vi "BinAndSaveWaveformsASCII.vi"(1 "transpose? (no:F)":bool, 4 "X step":dbl=0.10000000149011612 format="%.2f", 5 "format":string="%.6g", 6 "Deafault channel name prefix":string="CH", 7 "Channel name attribute":string="NI_ChannelName", 8 "error in":errorcluster, 9 "Save column names":bool, 10 "Y waveforms in":waveform(dbl)[](array[waveform]), 11 "file (use dialog)":path) -> (0 "error out":errorcluster)   [LabVIEW 2015]
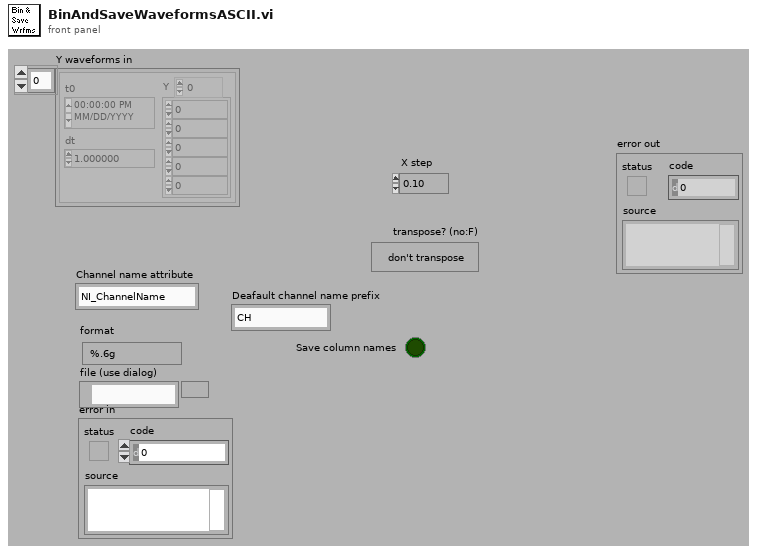
[diagram p1: front panel]
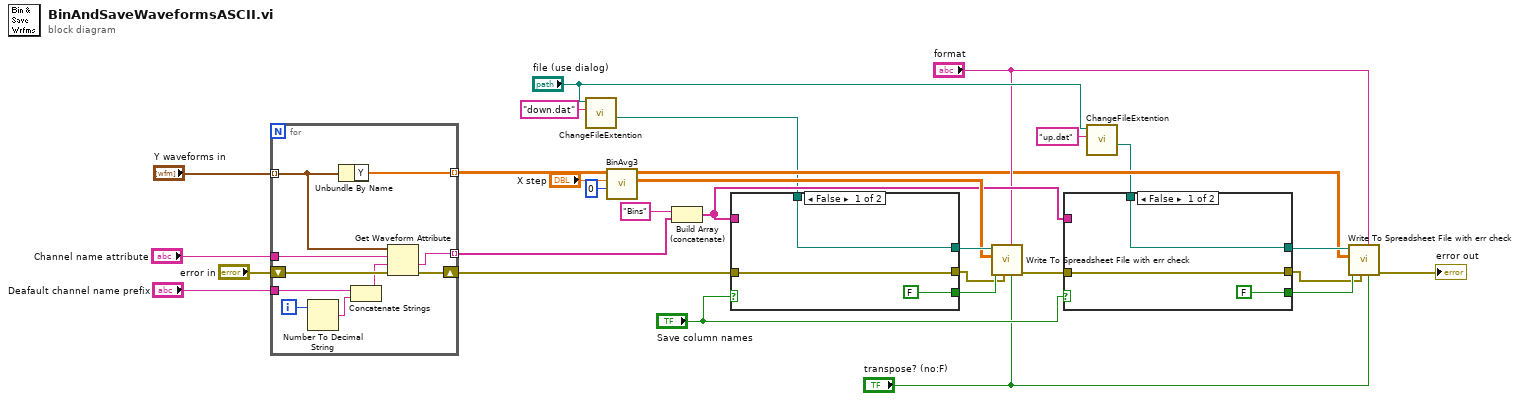
[diagram p0: block diagram]
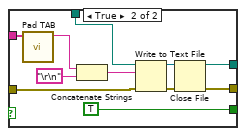
[diagram p2: hidden frame]
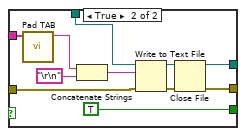
[diagram p3: hidden frame]
diagram:
  n1 = for {
    tunnel: "Y waveforms in" -> [w38] mode=indexing
    tunnel: [w39] -> w20 mode=indexing
    tunnel: "Channel name attribute" -> [w37]
    tunnel: "Deafault channel name prefix" -> [w36]
    shift-right: [w34] -> w22
    shift-left: "error in" -> [w35]
    tunnel: [w30] -> w23 mode=indexing
    i -> [w32]
    n2 = Number To Decimal String(number=w32) -> (decimal integer string=w31:string)  [unwired: 1 out]
    n3 = Unbundle By Name(w38) -> ("Y"=w39:dbl[])
    n4 = Concatenate Strings(w36, w31) -> (w33:string)
    n5 = Get Waveform Attribute(4:w35, 5:w33, 6:w37, 7:w38) -> (0:w34:errorcluster, 1:w30:string)  [unwired: 2 out]
  }
  n6 = call "ChangeFileExtention.vi"("New Extention"="down.dat", "Path"="file (use dialog)") -> ("Path with new extension"=w6:path)  [unwired: 1 in, 8 out]
  n7 = call "BinAvg3.vi"("X coumn index"=0 ("X column"), "Bin size"="X step", "Data in"=w20) -> ("Binned data down"=w17:dbl[][], "Binned data up"=w7:dbl[][])  [unwired: 1 in, 6 out]
  n8 = Build Array (concatenate)("Bins", w23) -> (w12:string[])
  n9 = case shown="False" "Save column names" {
    tunnel: [FALSE ("append to file? (new file:F)") TRUE] -> w28
    tunnel: [w40 w47] -> w27
    tunnel: w12 -> [_ w51]
    tunnel: [w41 w45] -> w26
    tunnel: w22 -> [w40 w44]
    tunnel: w6 -> [w41 w43]
    frame False {
    }
    frame True {
      n10 = call "Pad TAB.vi"("Input String Array"=w51) -> ("Output String"=w52:string)  [unwired: 1 in, 9 out]
      n11 = Concatenate Strings(w52, "\r\n") -> (w50:string)
      n12 = Write to Text File(file (use dialog)=w43, text=w50, error in=w44) -> (refnum out=w46:refnum<file>, error out=w48:errorcluster)  [unwired: 2 out]
      n13 = Close File(refnum=w46, error in=w48) -> (path=w45:path, error out=w47:errorcluster)
    }
  }
  n14 = call "Write To Spreadsheet File with err check.vi"("transpose? (no:F)"="transpose? (no:F)", "format (%.3f)"="format", "error in (no error)"=w27, "append to file? (new file:F)"=w28, "2D data"=w17, "file path (dialog if empty)"=w26) -> ("error out"=w11:errorcluster)  [unwired: 2 in, 3 out]
  n15 = call "ChangeFileExtention.vi"("New Extention"="up.dat", "Path"="file (use dialog)") -> ("Path with new extension"=w5:path)  [unwired: 1 in, 8 out]
  n16 = case shown="False" "Save column names" {
    tunnel: [FALSE ("append to file? (new file:F)") TRUE] -> w16
    tunnel: [w54 w61] -> w15
    tunnel: w12 -> [_ w65]
    tunnel: [w55 w59] -> w14
    tunnel: w11 -> [w54 w58]
    tunnel: w5 -> [w55 w57]
    frame False {
    }
    frame True {
      n17 = call "Pad TAB.vi"("Input String Array"=w65) -> ("Output String"=w66:string)  [unwired: 1 in, 9 out]
      n18 = Concatenate Strings(w66, "\r\n") -> (w64:string)
      n19 = Write to Text File(file (use dialog)=w57, text=w64, error in=w58) -> (refnum out=w60:refnum<file>, error out=w62:errorcluster)  [unwired: 2 out]
      n20 = Close File(refnum=w60, error in=w62) -> (path=w59:path, error out=w61:errorcluster)
    }
  }
  n21 = call "Write To Spreadsheet File with err check.vi"("transpose? (no:F)"="transpose? (no:F)", "format (%.3f)"="format", "error in (no error)"=w15, "append to file? (new file:F)"=w16, "2D data"=w7, "file path (dialog if empty)"=w14) -> ("error out"=→"error out":errorcluster)  [unwired: 2 in, 3 out]
